vi "setSelectedSheet.vi"(8 "error in (no error)":errorcluster, 10 "Sheet Ref":refnum<k24>, 11 "MS-Excel in":refnum<class "MS-Excel.lvclass">) -> (0 "error out":errorcluster, 3 "MS-Excel out":refnum<class "MS-Excel.lvclass">)   [LabVIEW 2017, in "LabVIEW NPOI.lvlib" / "MS-Excel.lvclass"]
uses:
  MS-Excel.lvclass
  C:/Users/Neo/Desktop/Dev_Tools_BR/LabVIEW_NPOI/src/lib/NPOI 2.1.1/NPOI.dll
  lib/NPOI 2.1.1/NPOI.dll
  MS-Excel.lvclass/MS-Excel.ctl
  <vilib>/Utility/error.llb/Error Cluster From Error Code.vi
  <vilib>/ErrorRing/Error Ring.xnode
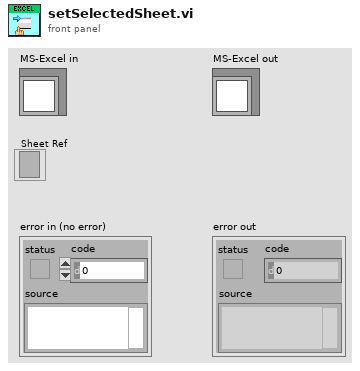
[diagram p1: front panel]
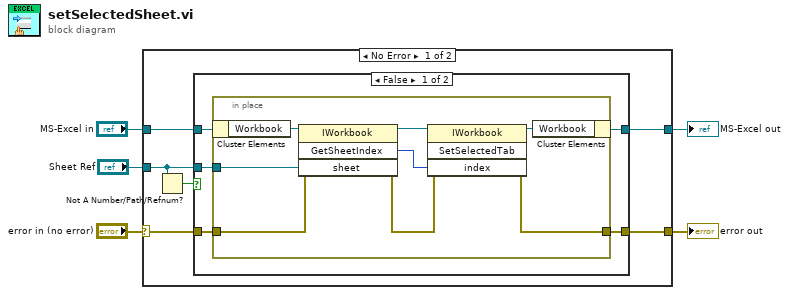
[diagram p0: block diagram]
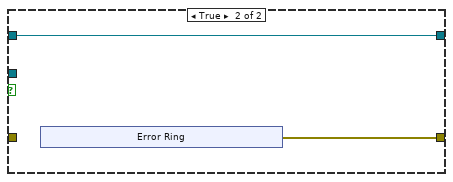
[diagram p2: hidden frame]
diagram:
  n1 = case shown="No Error" "error in (no error)" {
    selector: "error in (no error)" -> [w9 w31]
    tunnel: [w8 w31] -> w5
    tunnel: [w11 w32] -> w3
    tunnel: "MS-Excel in" -> [w10 w32]
    tunnel: "Sheet Ref" -> [w6 _]
    frame No Error {
      n2 = Not A Number/Path/Refnum?(number/path/refnum=w6) -> (NaN/Path/Refnum?=w7:bool)
      n3 = case shown="False" w7 {
        tunnel: [w16 w26] -> w11
        tunnel: w10 -> [w15 w26]
        tunnel: w9 -> [w14 _]
        tunnel: [w13 w25] -> w8
        tunnel: w6 -> [w12 _]
        frame False {
          n4 = in-place {
            in-place-border: w14 -> [w18]
            in-place-border: [w20] -> w13
            in-place-border: w12 -> [w17]
            n5 = in-place-cluster #1(w15) -> ("Workbook"=w22:refnum<k24>)
            n6 = invoke class="IWorkbook" method="GetSheetIndex"(reference=w22, error in=w18, "sheet"=w17) -> (reference out=w24:refnum<k24>, error out=w19:errorcluster, "GetSheetIndex"=w23:i32)  [unwired: 1 in, 1 out]
            n7 = invoke class="IWorkbook" method="SetSelectedTab"(reference=w24, error in=w19, "index"=w23) -> (reference out=w21:refnum<k24>, error out=w20:errorcluster)  [unwired: 1 in, 2 out]
            n8 = in-place-cluster #1("Workbook"=w21) -> (w16:refnum<class "MS-Excel.lvclass">)
          }
        }
        frame True {
          n9 = xnode "Error Ring"() -> ("error out"=w25:errorcluster)
        }
      }
    }
    frame Error {
    }
  }
  "error out" <- w5
  "MS-Excel out" <- w3
